vi "Write FSM Queue.vi"(8 "error in (no error)":errorcluster, 11 "App_State":T1=enum."App_Close") -> (0 "error out":errorcluster)   [LabVIEW 2017]
doc: "Enqueues a request for an application FSM state change."
uses:
  FSM States.ctl
  Application Globals.vi
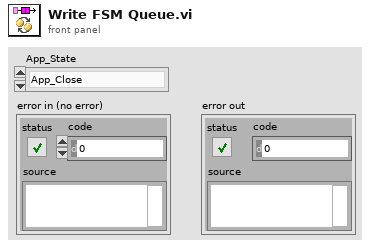
[diagram p1: front panel]
types:
  T1 = typedef "FSM States.ctl" = enum16{"App_Disconnect", "App_Idle", "App_Connect", "App_Close", "APP_Init", "App_Logging", "App_SetRecordStateOn", "App_SetRecordStateOff"}
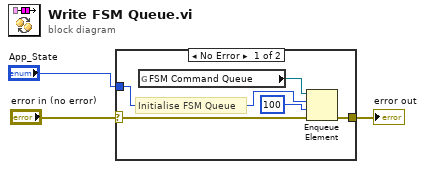
[diagram p0: block diagram]
diagram:
  n1 = case shown="No Error" "error in (no error)" {
    selector: "error in (no error)" -> [w6 w9]
    tunnel: [w5 w9] -> w3
    tunnel: "App_State" -> [w4 _]
    frame No Error {
      # "Initialise FSM Queue"
      n2 = global read "Application Globals.vi" "FSM Command Queue"() -> (w8:refnum<queue>)
      n3 = Enqueue Element(queue=w8, element=w4, timeout in ms (-1)=100, error in (no error)=w6) -> (error out=w5:errorcluster)  [unwired: 2 out]
    }
    frame Error {
    }
  }
  "error out" <- w3
